vi "Pack Auto-Launch Models Msg.vi"(6 "Confirm Shutdown? (T)":bool=TRUE, 9 "Auto-stop? (T)":bool=TRUE, 10 "Models":refnum<class "IModel.lvclass">[](array[class])) -> (3 "Launch Nested Models Msg":refnum<class "Auto-Launch Models Msg.lvclass">)   [LabVIEW 2019, in "IModel.lvlib" / "Auto-Launch Models Msg.lvclass"]
uses:
  <vilib>/gpm_packages/@cs/mva-core/Source/IModel/IModel Messages/Auto-Launch Models Msg/Auto-Launch Models Msg.lvclass
  <vilib>/gpm_packages/@cs/mva-core/Source/IModel/IModel/IModel.lvclass
  C:/Program Files/National Instruments/LabVIEW 2019/vi.lib/ActorFramework/Actor/Actor.lvclass
  <vilib>/gpm_packages/@cs/mva-core/Source/IModel/IModel Messages/Auto-Launch Models Msg/Auto-Launch Models Msg.lvclass/Auto-Launch Models Msg.ctl
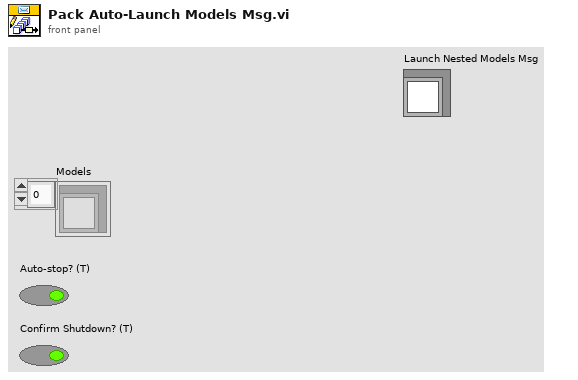
[diagram p1: front panel]
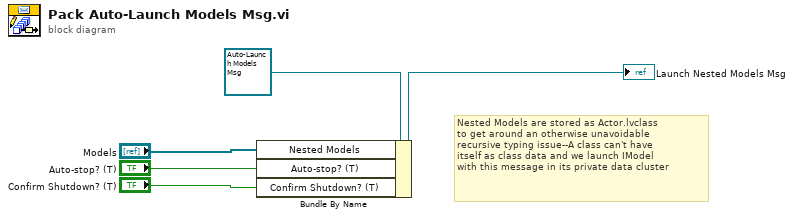
[diagram p0: block diagram]
diagram:
  # "Nested Models are stored as Actor.lvclass\nto get around an otherwise unavoidable\nrecursive typing issue--A class can't have\nitself as class data and we launch IModel\nwith this message in its private data cluster"
  n1 = Bundle By Name(cluster=refnum<class "Auto-Launch Models Msg.lvclass"> refnum ("Launch Nested Models Msg"), "Nested Models"="Models", "Auto-stop? (T)"="Auto-stop? (T)", "Confirm Shutdown? (T)"="Confirm Shutdown? (T)") -> (→"Launch Nested Models Msg":refnum<class "Auto-Launch Models Msg.lvclass">)
